vi "emi_Calculate polynomial.vi"(7 "X":dbl, 9 "Polly":dbl[](array[numeric])) -> (8 "Result":dbl)   [LabVIEW 2010]
doc: "Calkculates:\n\nResult = Poly[0] + x * Poly[1]+ x^2 * Poly[2] + x^3 * Poly[3] + x^4 * Poly[4] + x^5 * Poly[5] ....\nThe number of polynomials can be infinate. Efficiancy has proven to be quite good compared to direct hardcoding of specific polynomials(tests given 10000000 calculations of 4 polynomials = 95 ms vs a direct coding giving 55ms). The more polynomials the more efficient. This vi uses spesial cases for everything below four. Making it interchangable with a dedicated calculation.\n\nReentrant Subrouting. (reentrancy for improved eficiency only)"
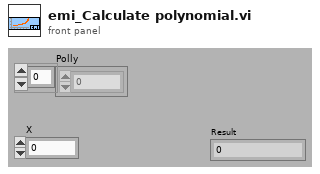
[diagram p1: front panel]
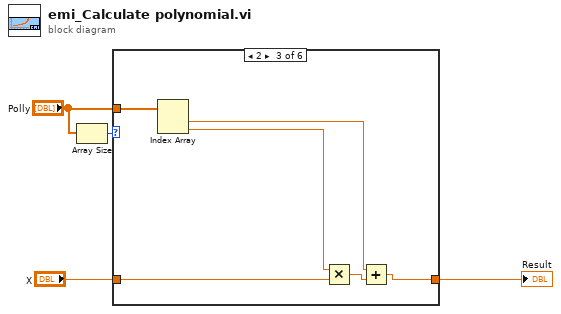
[diagram p0: block diagram]
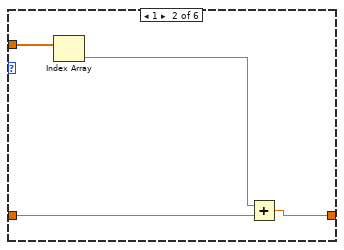
[diagram p3: hidden frame]
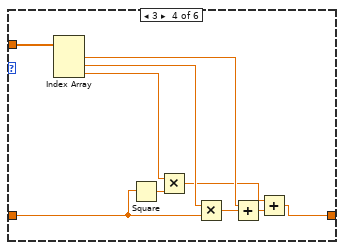
[diagram p4: hidden frame]
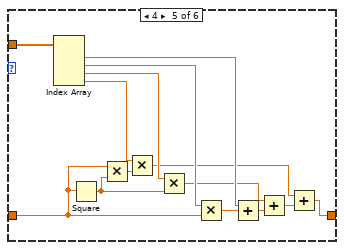
[diagram p5: hidden frame]
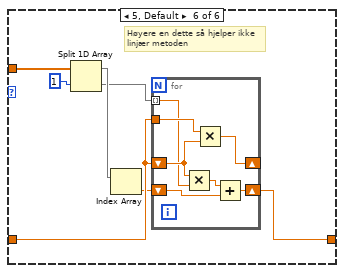
[diagram p6: hidden frame]
diagram:
  n1 = Array Size(array="Polly") -> (size(s)=w1:i32)
  n2 = case shown="2" w1 {
    tunnel: "X" -> [w5 w8 w12 w20 w31 w46]
    tunnel: [w5 w6 w13 w17 w27 w41] -> w3
    tunnel: "Polly" -> [_ w9 w15 w25 w39 w40]
    frame 0 {
    }
    frame 1 {
      n3 = Index Array(array=w9) -> (element=w7:dbl)  [unwired: 1 in]
      n4 = Add(x=w7, y=w8) -> (x+y=w6:dbl)
    }
    frame 2 {
      n5 = Index Array(array=w15) -> (element #1=w14:dbl, element #2=w11:dbl)  [unwired: 2 in]
      n6 = Multiply(x=w11, y=w12) -> (x*y=w10:dbl)
      n7 = Add(x=w14, y=w10) -> (x+y=w13:dbl)
    }
    frame 3 {
      n8 = Index Array(array=w25) -> (element #1=w24:dbl, element #2=w22:dbl, element #3=w18:dbl)  [unwired: 3 in]
      n9 = Square(x=w20) -> (x^2=w19:dbl)
      n10 = Multiply(x=w18, y=w19) -> (x*y=w16:dbl)
      n11 = Multiply(x=w22, y=w20) -> (x*y=w21:dbl)
      n12 = Add(x=w24, y=w21) -> (x+y=w23:dbl)
      n13 = Add(x=w16, y=w23) -> (x+y=w17:dbl)
    }
    frame 4 {
      n14 = Index Array(array=w39) -> (element #1=w38:dbl, element #2=w36:dbl, element #3=w34:dbl, element #4=w28:dbl)  [unwired: 4 in]
      n15 = Square(x=w31) -> (x^2=w30:dbl)
      n16 = Multiply(x=w31, y=w30) -> (x*y=w29:dbl)
      n17 = Multiply(x=w28, y=w29) -> (x*y=w26:dbl)
      n18 = Multiply(x=w34, y=w30) -> (x*y=w32:dbl)
      n19 = Multiply(x=w36, y=w31) -> (x*y=w35:dbl)
      n20 = Add(x=w38, y=w35) -> (x+y=w37:dbl)
      n21 = Add(x=w32, y=w37) -> (x+y=w33:dbl)
      n22 = Add(x=w26, y=w33) -> (x+y=w27:dbl)
    }
    frame 5, Default {
      # "Høyere en dette så hjelper ikke \nlinjær metoden"
      n23 = Split 1D Array(array=w40, index=1) -> (first subarray=w44:dbl[], second subarray=w43:dbl[])
      n24 = Index Array(array=w44) -> (element=w45:dbl)  [unwired: 1 in]
      n25 = for {
        tunnel: w43 -> [w50] mode=indexing
        tunnel: w46 -> [w53]
        shift-right: [w52] -> _
        shift-left: w46 -> [w51]
        shift-right: [w48] -> w41
        shift-left: w45 -> [w47]
        n26 = Multiply(x=w51, y=w50) -> (x*y=w49:dbl)
        n27 = Multiply(x=w53, y=w51) -> (x*y=w52:dbl)
        n28 = Add(x=w49, y=w47) -> (x+y=w48:dbl)
      }
    }
  }
  "Result" <- w3
